vi "FitGaussian1D.vi"(7 "1D Array to Fit":dbl[](array[numeric])) -> (4 "Best Gaussian Fit Array":dbl[](array[numeric]), 6 "Fit Amplitude":dbl, 8 "Fit Center":dbl, 10 "Fit 4*Sigma Width":dbl, 15 "Fit Offset":dbl)   [LabVIEW 2014]
uses:
  <vilib>/Analysis/NI_AALPro.lvlib
panel:
  out "error":i32
  in  "Initial Guess":T1={"initial amplitude"=nan, "initial center"=nan, "initial standard deviation"=nan, "offset"=nan}
  out "Automatic Guess":cluster{dbl, i32, dbl, dbl}
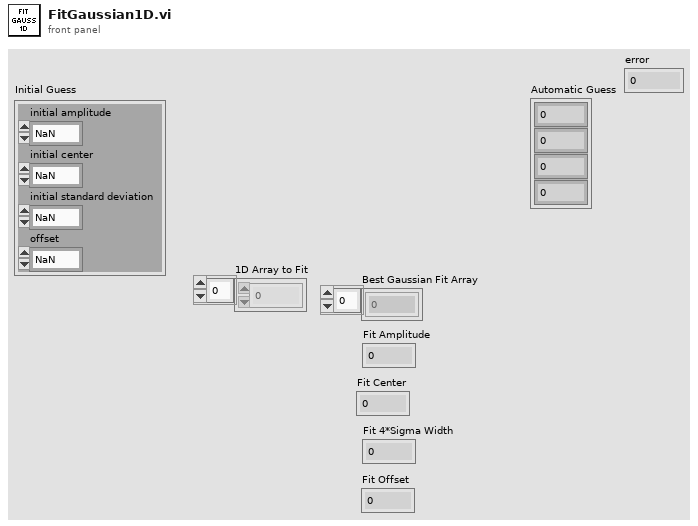
[diagram p1: front panel]
types:
  T1 = cluster{"initial amplitude":dbl, "initial center":dbl, "initial standard deviation":dbl, "offset":dbl}
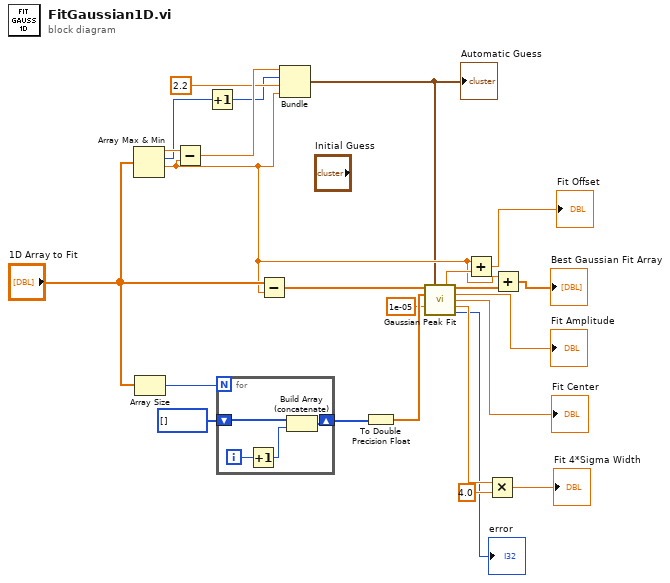
[diagram p0: block diagram]
diagram:
  n1 = Array Max & Min(array="1D Array to Fit") -> (max value=w22:dbl, max index (indices)=w19:i32, min value=w7:dbl)  [unwired: 1 out]
  n2 = Array Size(array="1D Array to Fit") -> (size(s)=w24:i32)
  n3 = Subtract(x=w22, y=w7) -> (x-y=w21:dbl)
  n4 = Increment(x=w19) -> (x+1=w18:i32)
  n5 = for {
    N: w24 -> [_]
    shift-right: [w27] -> w5
    shift-left: i32[] [] -> [w28]
    i -> [w26]
    n6 = Increment(x=w26) -> (x+1=w25:i32)
    n7 = Build Array (concatenate)(w28, w25) -> (w27:i32[])
  }
  n8 = Subtract(x="1D Array to Fit", y=w7) -> (x-y=w11:dbl[])
  n9 = Bundle(w21, w18, 2.2, w7) -> (w1:cluster{dbl, i32, dbl, dbl})  [unwired: 1 in]
  "Automatic Guess" <- w1
  n10 = To Double Precision Float(number=w5) -> (double precision float=w4:dbl[])
  n11 = call <vilib>:"Gaussian Peak Fit.vi"("Y"=w11, "initial guess"=w1, "X"=w4, "tolerance"=1e-05) -> ("offset"=w10:dbl, "Best Gaussian Fit"=w8:dbl[], "amplitude"=→"Fit Amplitude":dbl, "center"=→"Fit Center":dbl, "standard deviation"=w15:dbl, "error"=→"error":i32)  [unwired: 5 in, 1 out]
  n12 = Add(x=w7, y=w10) -> (x+y=→"Fit Offset":dbl)
  n13 = Multiply(x=w15, y=4.0) -> (x*y=→"Fit 4*Sigma Width":dbl)
  n14 = Add(x=w7, y=w8) -> (x+y=→"Best Gaussian Fit Array":dbl[])
